vi "Post Event.vi"(7 "Tag":T1, 8 "error in (no error)":errorcluster caption="错误输入（无错误）", 9 "Event Data":variant, 10 "Event Name":string, 11 "User Event Collection 输入":refnum<class "User Event Collection.lvclass"> caption="DNL_LabVIEW Object in") -> (0 "error out":errorcluster caption="错误输出", 3 "User Event Collection 输出":refnum<class "User Event Collection.lvclass"> caption="DNL_LabVIEW Object out")   [LabVIEW 2013, in "User Event Collection.lvclass"]
uses:
  User Event Collection.lvclass
  Tag.ctl
  User Event Collection.lvclass/User Event Collection.ctl
  <resource>/importtools/Common/Event/NISAST Event.lvclass
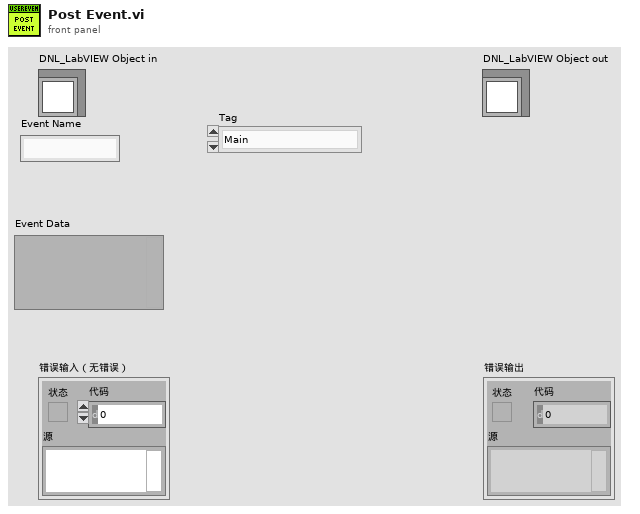
[diagram p1: front panel]
types:
  T1 = typedef "User Event Collection.lvclass/Tag.ctl" = enum16{"Main", "UI"}
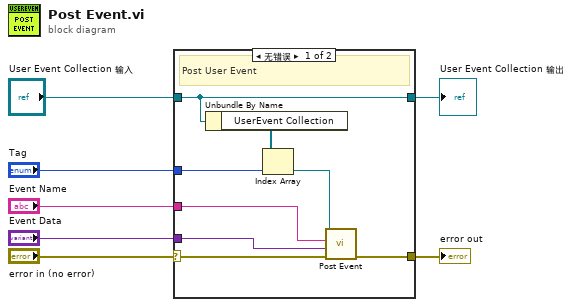
[diagram p0: block diagram]
diagram:
  n1 = case shown="无错误" "error in (no error)" {
    selector: "error in (no error)" -> [w9 w17]
    tunnel: [w8 w17] -> w6
    tunnel: [w15 w16] -> w4
    tunnel: "User Event Collection 输入" -> [w15 w16]
    tunnel: "Event Name" -> [w11 _]
    tunnel: "Event Data" -> [w10 _]
    tunnel: "Tag" -> [w13 _]
    frame No Error {
      # "Post User Event"
      n2 = Unbundle By Name(w15) -> ("UserEvent Collection"=w14:refnum<class "NISAST Event.lvclass">[])
      n3 = Index Array(array=w14, index=w13) -> (element=w12:refnum<class "NISAST Event.lvclass">)
      n4 = call-dynamic "Post Event.vi"("error in (no error)"=w9, "Event Data"=w10, "Event Name"=w11, "Event in"=w12) -> ("error out"=w8:errorcluster)  [unwired: 6 in, 1 out]
    }
    frame Error {
    }
  }
  "error out" <- w6
  "User Event Collection 输出" <- w4
